vi "FeedbackDecode_CompName2IP.vi"() -> (0 "CompID":T1={"LV"={"Name"="ClinicalLabview", "IP"=""}, "ML"={"Name"="ClinicalMatlab", "IP"=""}})   [LabVIEW 2016]
uses:
  <vilib>/regexp/Match Regular Expression.xnode
panel:
  out "standard output":string
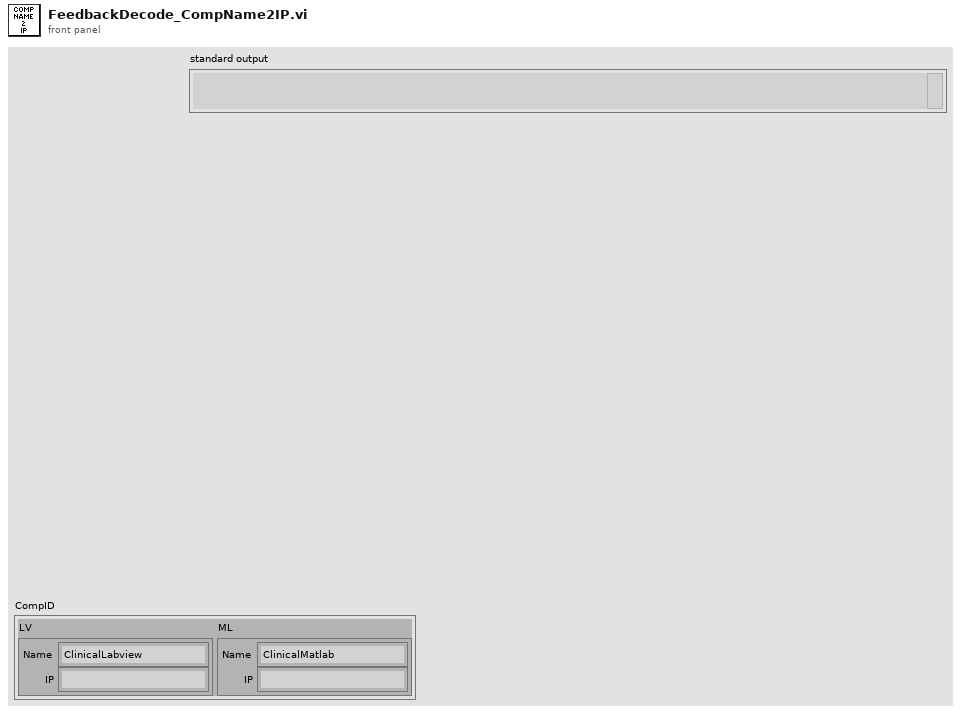
[diagram p1: front panel]
types:
  T1 = cluster{"LV":cluster{"Name":string, "IP":string}, "ML":cluster{"Name":string, "IP":string}}
  T2 = cluster{"[0]":cluster{"Name":string, "IP":string}, "[1]":cluster{"Name":string, "IP":string}}
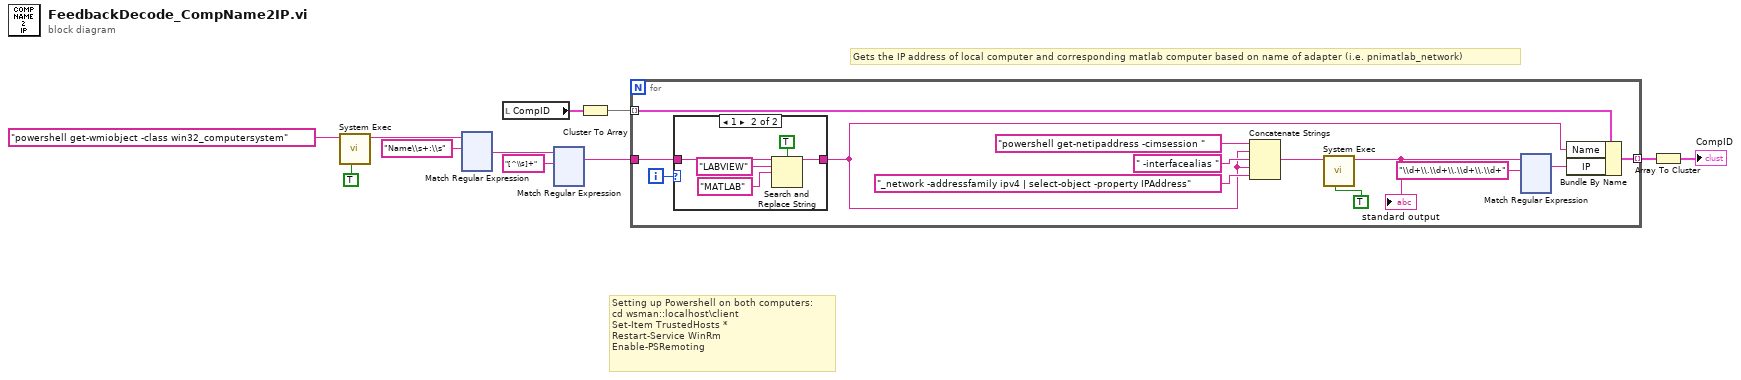
[diagram p0: block diagram]
diagram:
  # "Setting up Powershell on both computers:\ncd wsman::localhost\\client\nSet-Item TrustedHosts *\nRestart-Service WinRm\nEnable-PSRemoting"
  # "Gets the IP address of local computer and corresponding matlab computer based on name of adapter (i.e. pnimatlab_network)"
  n1 = call <vilib>:"System Exec.vi"("run minimized? (F)"=TRUE, "command line"="powershell get-wmiobject -class win32_computersystem") -> ("standard output"=w9:string)  [unwired: 6 in, 3 out]
  n2 = xnode "Match Regular Expression"("input string"=w9, "regular expression"="Name\\s+:\\s") -> ("after match"=w7:string)  [unwired: 4 in, 4 out]
  n3 = local read "CompID"() -> (w4:T1)
  n4 = xnode "Match Regular Expression"("input string"=w7, "regular expression"="[^\\s]+") -> ("whole match"=w3:string)  [unwired: 4 in, 4 out]
  n5 = Cluster To Array(cluster=w4) -> (array=w1:cluster{"Name":string, "IP":string}[])
  n6 = for {
    tunnel: w3 -> [w20]
    tunnel: [w17] -> w2 mode=indexing
    tunnel: w1 -> [w18] mode=indexing
    i -> [w21]
    n7 = case shown="1" w21 {
      tunnel: w20 -> [w25 w30]
      tunnel: [w25 w29] -> w13
      frame 0, Default {
      }
      frame 1 {
        n8 = Search and Replace String(case sensitive?=TRUE ("ignore case? (F)"), input string=w30, search string="LABVIEW", replace string="MATLAB" ("search string")) -> (result string=w29:string)  [unwired: 4 in, 3 out]
      }
    }
    n9 = Concatenate Strings("powershell get-netipaddress -cimsession " ("command line"), w13, " -interfacealias " ("command line"), w13, "_network -addressfamily ipv4 | select-object -property IPAddress" ("command line")) -> (w12:string)
    n10 = call <vilib>:"System Exec.vi"("run minimized? (F)"=TRUE, "command line"=w12) -> ("standard output"=w23:string)  [unwired: 6 in, 3 out]
    "standard output" <- w23
    n11 = xnode "Match Regular Expression"("input string"=w23, "regular expression"="\\d+\\.\\d+\\.\\d+\\.\\d+") -> ("whole match"=w19:string)  [unwired: 4 in, 4 out]
    n12 = Bundle By Name(cluster=w18, "Name"=w13, "IP"=w19) -> (w17:cluster{"Name":string, "IP":string})
  }
  n13 = Array To Cluster(array=w2) -> (cluster=→"CompID":T2)
